vi "maskOp (U16).vi"(1 "Mask":T1[](array[typedef]) items=["---", "OFF", "ON"], 2 "Original":u16) -> (0 "Result":u16)   [LabVIEW 2023, in "canopen.lvlib"]
doc: "Gets the flattened list of controls inside a specific container."
uses:
  canopen.lvlib
  types/threestateFlag.ctl
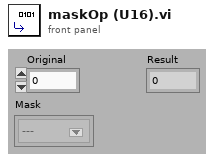
[diagram p1: front panel]
types:
  T1 = typedef "canopen.lvlib/threestateFlag.ctl" = i8
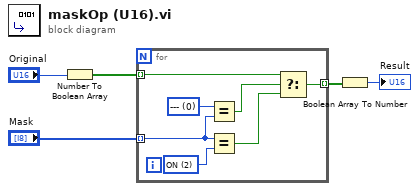
[diagram p0: block diagram]
diagram:
  n1 = Number To Boolean Array(number="Original") -> (Boolean array=w4:bool[])
  n2 = for {
    tunnel: w4 -> [w12] mode=indexing
    tunnel: "Mask" -> [w6] mode=indexing
    tunnel: [w11] -> w2 mode=indexing
    w10 = T1 2 items=["---", "OFF", "ON"] ("New value")
    w7 = T1 0 items=["---", "OFF", "ON"] ("New value")
    n3 = Equal?(x=w7, y=w6) -> (x = y?=w8:bool)
    n4 = Equal?(x=w6, y=w10) -> (x = y?=w9:bool)
    n5 = Select(t=w12, s=w8, f=w9) -> (s? t:f=w11:bool)
  }
  n6 = Boolean Array To Number(Boolean array=w2) -> (number=→"Result":u32)
